vi "Set_niLabel.vi"(8 "error in (no error)":errorcluster, 10 "data":T1, 11 "niLabel in":refnum<class "niLabel.lvclass">) -> (0 "error out":errorcluster, 3 "niLabel out":refnum<class "niLabel.lvclass">)   [LabVIEW 2020, in "niLabel.lvclass"]
uses:
  <vilib>/AppBuilder/IB_Classes/Destination/niLabel/niLabel.lvclass
  <vilib>/AppBuilder/IB_Classes/Destination/niLabel/niLabel.lvclass/niLabel.ctl
  <vilib>/AppBuilder/IB_Classes/Destination/niLabel/IB_Dest_niLabel.ctl
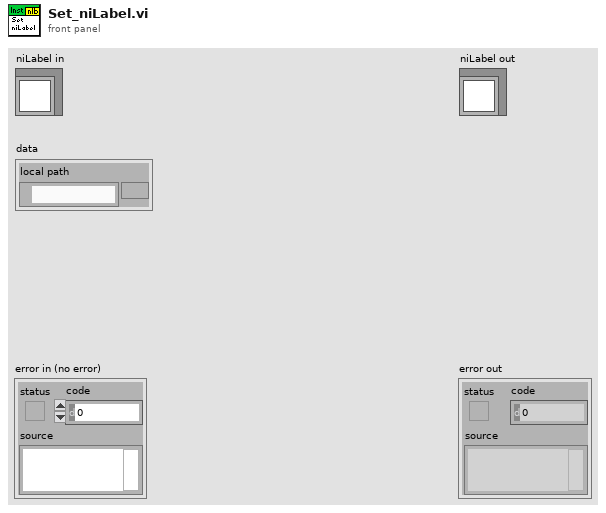
[diagram p1: front panel]
types:
  T1 = typedef "IB_Dest_niLabel.ctl" = cluster{"local path":path}
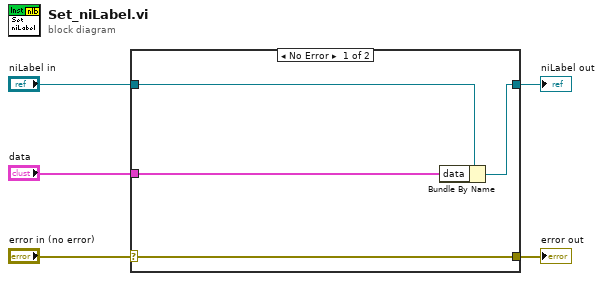
[diagram p0: block diagram]
diagram:
  n1 = case shown="No Error" "error in (no error)" {
    selector: "error in (no error)" -> [w9 w10]
    tunnel: [w9 w10] -> w4
    tunnel: [w7 w11] -> w2
    tunnel: "niLabel in" -> [w8 w11]
    tunnel: "data" -> [w6 _]
    frame No Error {
      n2 = Bundle By Name(cluster=w8, "data"=w6) -> (w7:refnum<class "niLabel.lvclass">)
    }
    frame Error {
    }
  }
  "error out" <- w4
  "niLabel out" <- w2
